vi "tagDB Proble.vi"(11 "DB Ref":T1) -> (2 "Value String":string, 3 "Boolean":bool)   [LabVIEW 2014]
uses:
  TagDB/tagDB_Def.ctl
  TagDB/TagDB(dev).lvlib
panel:
  out "Valid?":bool
  out "Name":string
  out "DataItemFlag":i64
  out "DataChangeFlag":i64
  in  "Items":i32(listbox)
  out "VI Server Type":T2(ring)=enum."VI"
  out "Data Type":T3(ring)
  out "data":variant
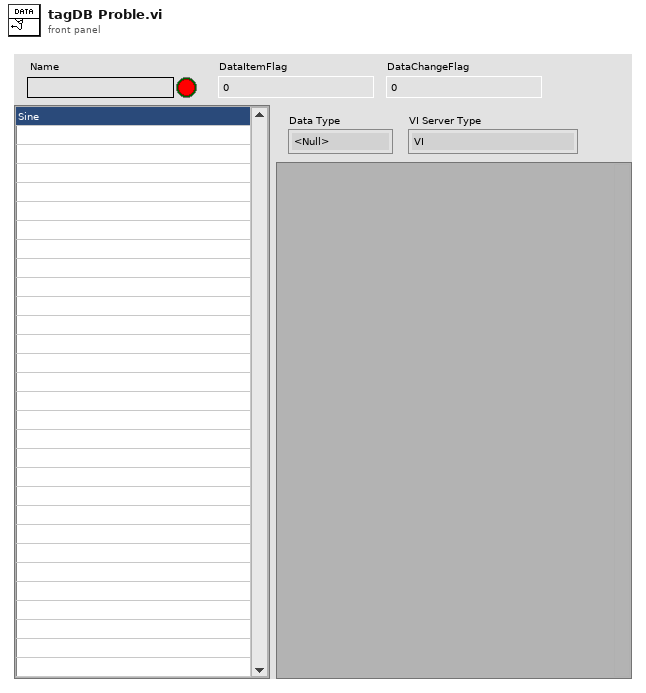
[diagram p1: front panel]
types:
  T1 = typedef "TagDB(dev).lvlib/tagDB_Def.ctl" = refnum<k1>
  T2 = enum16{"Not a VI Server Refnum", "Control", "VI", "Application", "Splitter", "Pane"}
  T3 = enum8{"<Null>", "I8", "I16", "I32", "I64", "U8", "U16", "U32", "U64", "SGL", "DBL", "EXT", "CSG", "CDB", "CXT", "0x0F", "0x10", "0x11", "0x12", "0x13", "0x14", "Enum U8", "Enum U16", "Enum U32", "Enum U64", "SGL PQ", "DBL PQ", "EXT PQ", "CSG PQ", "CDB PQ", "CXT PQ", "0x1F", "0x20", "Boolean", "0x22", "0x23", "0x24", "0x25", "0x26", "0x27", "0x28", "0x29", "0x2A", "0x2B", "0x2C", "0x2D", "0x2E", "0x2F", "String", "0x31", "Path", "Pict", "0x34", "0x35", "0x36", "DAQ", "0x38", "0x39", "0x3A", "0x3B", "0x3C", "0x3D", "0x3E", "0x3F", "Array", "0x41", "0x42", "0x43", "0x44", "0x45", "0x46", "0x47", "0x48", "0x49", "0x4A", "0x4B", "0x4C", "0x4D", "0x4E", "0x4F", "Cluster", "0x51", "0x52", "Variant", "Waveform", "0x55", "0x56", "0x57", "0x58", "0x59", "0x5A", "0x5B", "0x5C", "0x5D", "0x5E", "0x5F", "0x60", "0x61", "0x62", "0x63", "0x64", "0x65", "0x66", "0x67", "0x68", "0x69", "0x6A", "0x6B", "0x6C", "0x6D", "0x6E", "0x6F", "Refnum"}
  T4 = typedef "TagDB(dev).lvlib/_DEF-DATA.ctl" = cluster{"data hashmap":variant, "DataChangeFlag":i64, "ItemChangeFlag":i64, "name":string, "Tag Adding Lock?":bool}
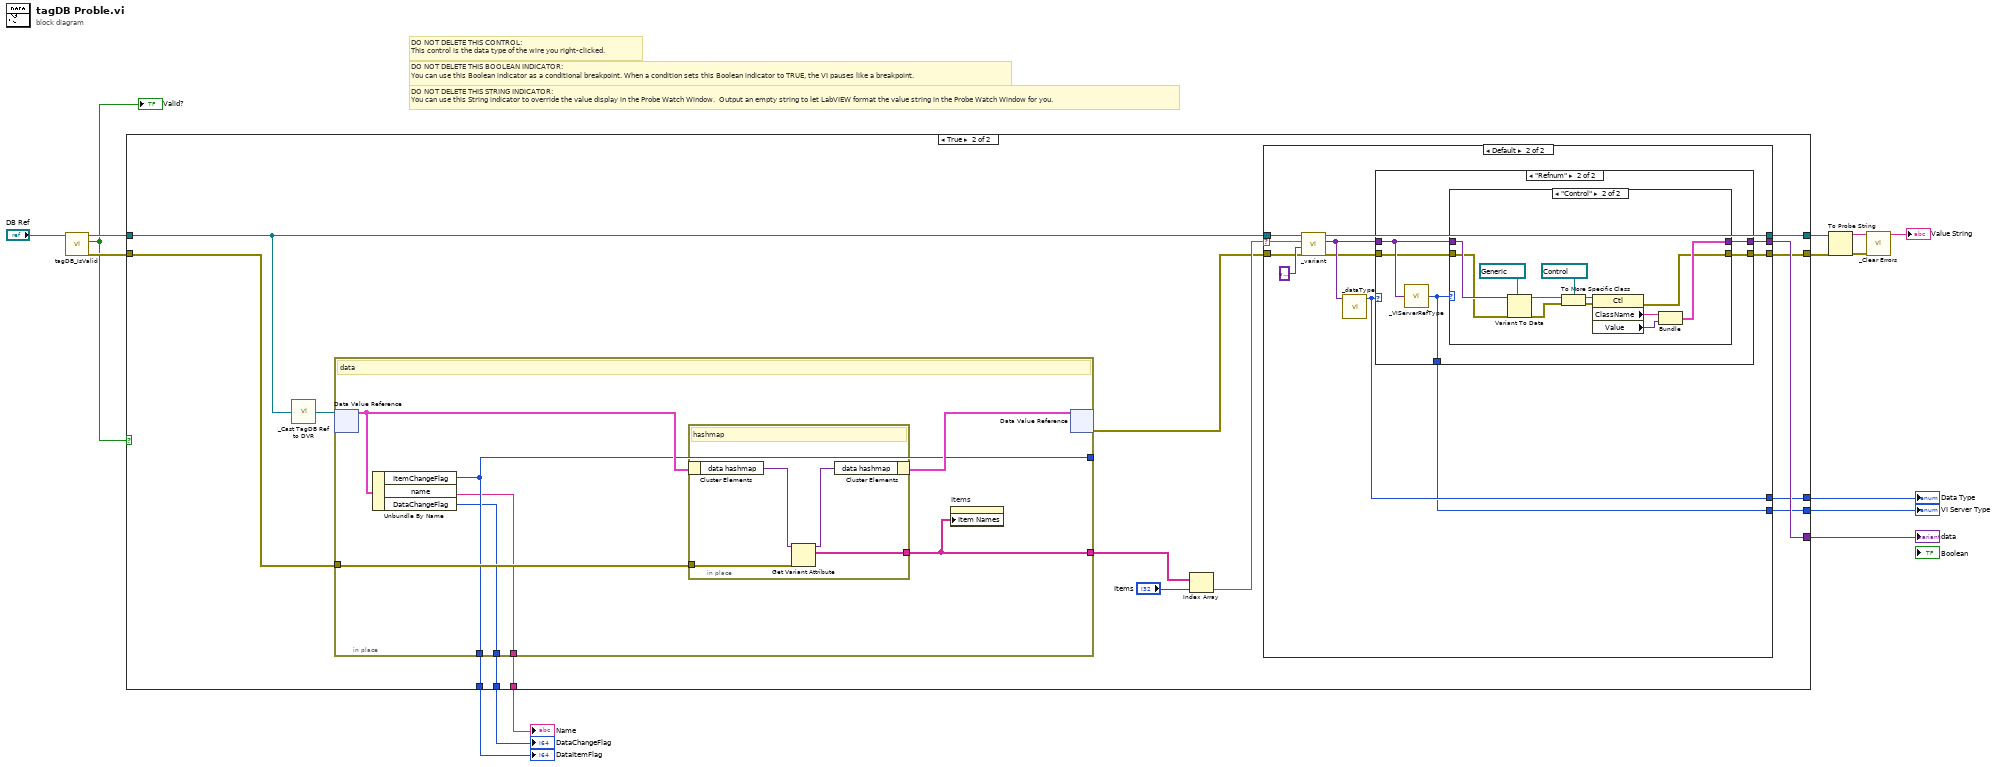
[diagram p0: block diagram]
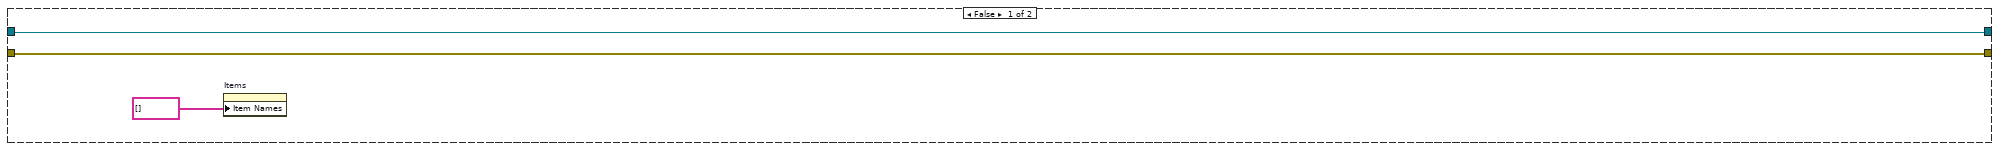
[diagram p2: hidden frame]
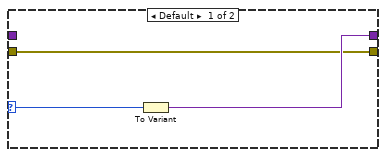
[diagram p5: hidden frame]
diagram:
  # "DO NOT DELETE THIS STRING INDICATOR: \nYou can use this String indicator to override the value display in the Probe Watch Window.  Output an empty string to let LabVIEW format the value string in the Probe Watch Window for you."
  # "DO NOT DELETE THIS BOOLEAN INDICATOR: \nYou can use this Boolean indicator as a conditional breakpoint. When a condition sets this Boolean indicator to TRUE, the VI pauses like a breakpoint."
  # "DO NOT DELETE THIS CONTROL: \nThis control is the data type of the wire you right-clicked."
  n1 = call "tagDB_IsValid.vi"("DB Ref in"="DB Ref") -> ("error out"=w10:errorcluster, "valid?"=w7:bool, "DB Ref out"=w11:T1)  [unwired: 8 in]
  "Valid?" <- w7
  n2 = case shown="True" w7 {
    tunnel: [_ w32] -> w12
    tunnel: w11 -> [w17 w31]
    tunnel: w10 -> [w16 w19]
    tunnel: [w17 w30] -> w9
    tunnel: [w16 w29] -> w8
    tunnel: [_ w24] -> w5
    tunnel: [_ w23] -> w4
    tunnel: [_ w22] -> w3
    tunnel: [_ w21] -> w2
    tunnel: [_ w20] -> w1
    frame False {
      n3 = property on="Items" class="LstBox (strict)"("Item Names"=string[] []) -> ()  [unwired: 2 in, 2 out]
    }
    frame True {
      n4 = call "_Cast TagDB Ref to DVR.vi"("TagDB"=w31) -> ("DVR"=w18:refnum<data-value>)  [unwired: 4 in]
      n5 = in-place {
        in-place-border: [w38] -> w28
        in-place-border: [w35] -> _
        in-place-border: w19 -> [w36]
        in-place-border: [w35] -> w22
        in-place-border: [w34] -> w21
        in-place-border: [w33] -> w20
        # "data"
        n6 = in-place-dvr #1(w18) -> (w37:T4)  [unwired: 1 out]
        n7 = Unbundle By Name(w37) -> ("ItemChangeFlag"=w35:i64, "name"=w33:string, "DataChangeFlag"=w34:i64)
        n8 = in-place {
          in-place-border: [w41] -> w38
          in-place-border: w36 -> [w40]
          # "hashmap"
          n9 = in-place-cluster #2(w37) -> ("data hashmap"=w43:variant)
          n10 = Get Variant Attribute(Variant=w43, error in=w40) -> (duplicate Variant=w42:variant, names=w41:string[])  [unwired: 2 in, 2 out]
          n11 = in-place-cluster #2("data hashmap"=w42) -> (w39:T4)
        }
        n12 = property on="Items" class="LstBox (strict)"("Item Names"=w38) -> ()  [unwired: 2 in, 2 out]
        n13 = in-place-dvr #1(w39) -> (w25:errorcluster)  [unwired: 1 out]
      }
      n14 = Index Array(array=w28, index="Items") -> (element=w26:string)
      n15 = case shown="Default" w26 {
        selector: w26 -> [_ w55]
        tunnel: w31 -> [w45 w56]
        tunnel: [w45 w54] -> w30
        tunnel: [w44 w48] -> w29
        tunnel: [_ w51] -> w32
        tunnel: w25 -> [w44 w52]
        tunnel: [_ w47] -> w24
        tunnel: [_ w46] -> w23
        frame "" {
        }
        frame Default {
          n16 = call "_variant.vi"("error in (no error)"=w52, "default value (empty variant)"=variant, "name"=w55, "DB Ref"=w56) -> ("error out"=w49:errorcluster, "value"=w50:variant, "DB Ref (dup)"=w54:T1)  [unwired: 5 in]
          n17 = call "_dataType.vi"("Type"=w50) -> ("type"=w47:T3)  [unwired: 10 in]
          n18 = case shown="\"Refnum\"" w47 {
            tunnel: [w58 w63] -> w51
            tunnel: w50 -> [w58 w62]
            tunnel: w49 -> [w57 w61]
            tunnel: [w57 w60] -> w48
            tunnel: [_ w59] -> w46
            frame Default {
            }
            frame "Refnum" {
              n19 = call "_VIServerRefType.vi"("Data"=w62) -> ("Enum"=w59:T2)  [unwired: 4 in]
              n20 = case shown="\"Control\"" w59 {
                selector: w59 -> [w66 _]
                tunnel: [w65 w69] -> w63
                tunnel: w62 -> [_ w78]
                tunnel: w61 -> [w64 w68]
                tunnel: [w64 w67] -> w60
                frame Default {
                  n21 = To Variant(anything=w66) -> (Variant=w65:variant)
                }
                frame "Control" {
                  n22 = Variant To Data(error in=w68, type=refnum<vi> refnum ("value"), Variant=w78) -> (data=w76:refnum<vi>, error out=w75:errorcluster)
                  n23 = To More Specific Class(target class=refnum<vi> refnum ("value"), reference=w76, error in=w75) -> (specific class reference=w73:refnum<vi>, error out=w72:errorcluster)
                  n24 = property class="Ctl"(reference=w73, error in=w72) -> (error out=w67:errorcluster, "ClassName"=w71:string, "Value"=w70:variant)  [unwired: 1 out]
                  n25 = Bundle("ClassName"=w71, "Value"=w70) -> (w69:cluster{"ClassName":string, "Value":variant})  [unwired: 1 in]
                }
              }
            }
          }
        }
      }
    }
  }
  "data" <- w12
  "Data Type" <- w5
  "VI Server Type" <- w4
  "DataChangeFlag" <- w2
  "DataItemFlag" <- w3
  "Name" <- w1
  n26 = To Probe String(4:w8, 7:w9) -> (0:w6:errorcluster, 3:→"Value String":string)  [unwired: 1 in]
  n27 = call "_Clear Errors.vi"("error in (no error)"=w6) -> ()  [unwired: 5 in, 2 out]
